vi "UI_visual2.vi"() -> ()   [LabVIEW 2017]
uses:
  <vilib>/picture/3D Picture Control/NI_3D Picture Control.lvlib
  <vilib>/picture/3D Picture Control/Object/Add Object (no reference).vi
  <vilib>/Utility/miscctls.llb/LV3DPointTypeDef.ctl
  <vilib>/Analysis/coordinate.llb/Euler Rotation Order.ctl
  <vilib>/Analysis/NI_AALPro.lvlib
  <vilib>/picture/3D Picture Control/Object/Create Object (name).vi
  <vilib>/picture/3D Picture Control/Helpers/Apply Texture (no reference).vi
  <vilib>/picture/3D Picture Control/Helpers/Set Clip Plane (no reference).vi
panel:
  out "element":dbl
  in  "Simulation Parameters":T1={"Wind VelocityAzimuth [deg] "=0.0, "Wind Velocity Module [m/s]"=0.0, "Fe gain"=1.0, "Cnalpha gain"=1.0, "clp gain"=1.0, "cld gain"=1.0, "cmq gain"=1.0, "cnr gain"=1.0, "dl [º]"=0.0, "Nozzle misalignment yaw/pitch [º]"=[0.0, 0.0], "Nozzle eccentricity x/y [m]"=[], "Wind_Profile"=0} {"Wind_Profile" min=0 max=3 step=1; "Wind Velocity Module [m/s]" format="%#_13g"; "Wind VelocityAzimuth [deg]" format="%#_13g"}
  in  "Initialization Parameters":T2={"W_b ini [rad/s]"=[0.0, 0.0, 0.0], "W ini [rad/s]"=[0.0, 0.0, 0.0], "altitude_ini(m)"=50.0, "lon_ini [º]"=-44.36778, "latd_ini [º]"=-2.31599, "V_ini [m/s]"=[0.0, 0.0, 0.0], "Initial Euler Angles [deg]"=[0.0, 0.0, 0.0], "CFN-61G Enable"=FALSE, "Table enable"=FALSE, "DMARS Enable"=FALSE, "TVA Enable"=FALSE, "Sim_Time [s]"=82.0}
  out "CRC data fault":bool
  out "Euler Angles [rad]":dbl[](array[numeric])
  in  "Tab Control":T3(tab)
  out "Position":cluster{dbl[], dbl[]}[](graph)
  out "Velocity":cluster{dbl[], dbl[]}[](graph)
  out "Quaternions":cluster{dbl[], dbl[]}[](graph)
  out "Euler Angles":cluster{dbl[], dbl[]}[](graph)
  out "Body Rates":cluster{dbl[], dbl[]}[](graph)
  out "Body Accelerations":cluster{dbl[], dbl[]}[](graph)
  out "Malpha/ Mbeta":cluster{dbl[], dbl[]}[](graph)
  out "Angles of attack":cluster{dbl[], dbl[]}[](graph)
  out "ACT_b_angles":cluster{dbl[], dbl[]}[](graph)
  out "Oil Consumption":cluster{dbl[], dbl[]}(graph)
  out "Bending Moments":dbl[](graph)
  out "CRC Failures":cluster{dbl[], dbl[]}[](graph)
  out "Euler Angles 2":cluster{dbl[], dbl[]}[](graph)
  out "Sim_Stopped":bool
  in  "stop Host":bool
  in  "Run_SIM":bool
  out "time[s]":dbl
  out "Euler Angles [º]":dbl[](array[numeric])
  out "B-frame [m]":cluster{"X":sgl, "Y":sgl, "Z":sgl}
  in  "B-frame Translation 2":cluster{"X":sgl, "Y":sgl, "Z":sgl}
  in  "N-frame rot":dbl[](array[numeric])
  in  "Up Direction":T4={"X"=0.0, "Y"=0.0, "Z"=1.0}
  out "3D Picture Control":refnum<vi>(3d-picture)
  in  "error in (no error)":errorcluster
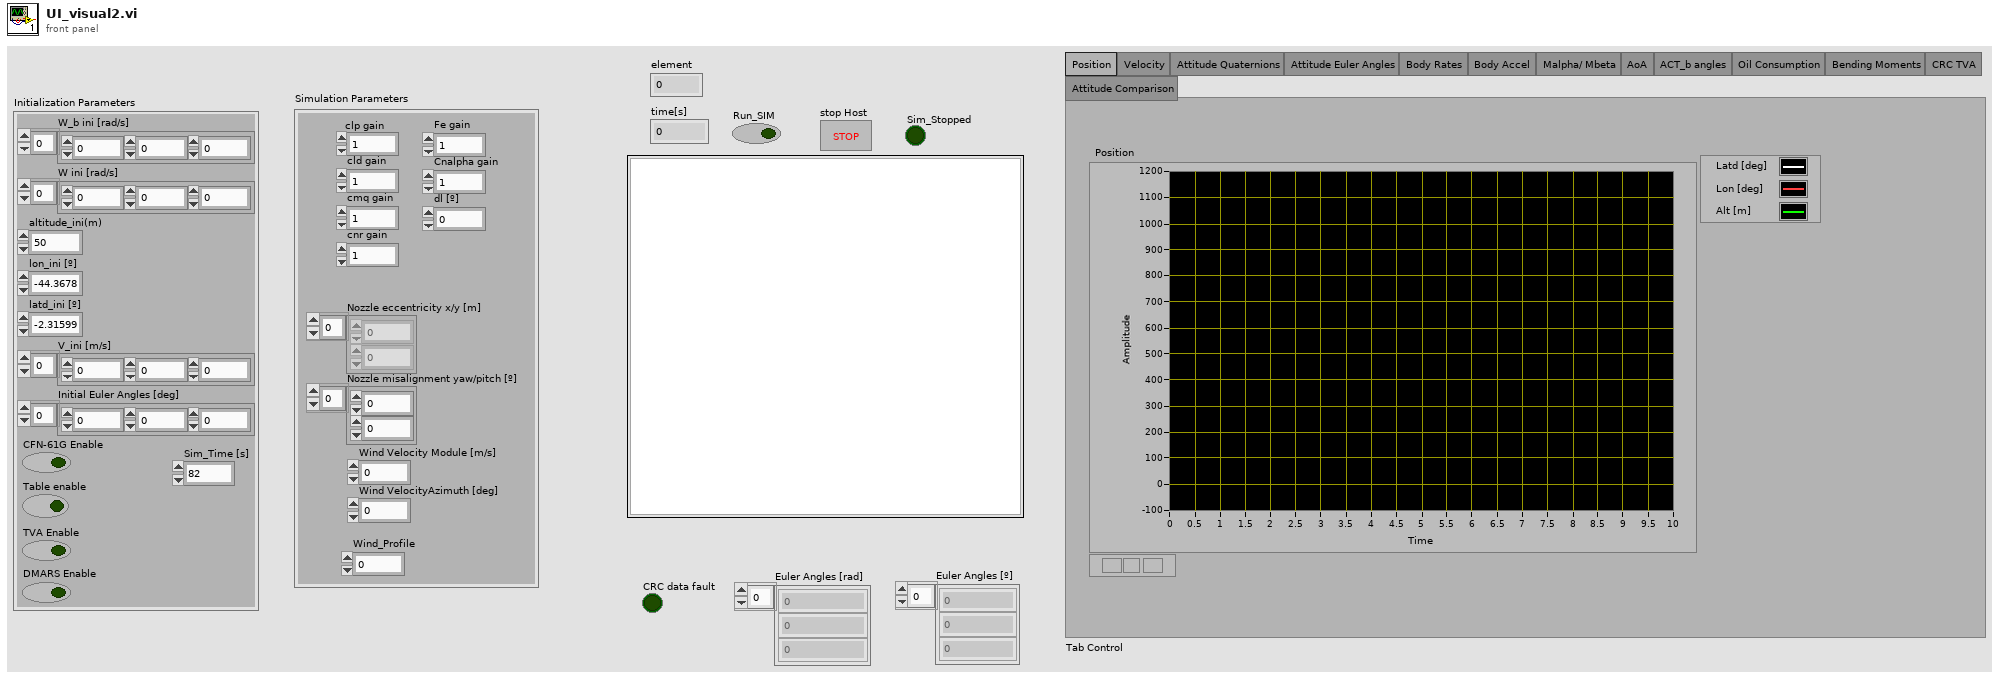
[diagram p1: front panel]
types:
  T1 = cluster{"Wind VelocityAzimuth [deg] ":dbl, "Wind Velocity Module [m/s]":dbl, "Fe gain":dbl, "Cnalpha gain":dbl, "clp gain":dbl, "cld gain":dbl, "cmq gain":dbl, "cnr gain":dbl, "dl [º]":dbl, "Nozzle misalignment yaw/pitch [º]":dbl[], "Nozzle eccentricity x/y [m]":dbl[], "Wind_Profile":i32}
  T2 = cluster{"W_b ini [rad/s]":dbl[], "W ini [rad/s]":dbl[], "altitude_ini(m)":dbl, "lon_ini [º]":dbl, "latd_ini [º]":dbl, "V_ini [m/s]":dbl[], "Initial Euler Angles [deg]":dbl[], "CFN-61G Enable":bool, "Table enable":bool, "DMARS Enable":bool, "TVA Enable":bool, "Sim_Time [s]":dbl}
  T3 = enum32{"Position", "Velocity", "Attitude Quaternions", "Attitude Euler Angles", "Body Rates", "Body Accel", "Malpha/ Mbeta", "AoA", "ACT_b angles", "Oil Consumption", "Bending Moments", "CRC TVA", "Attitude Comparison"}
  T4 = typedef "LV3DPointTypeDef.ctl" = cluster{"X":sgl, "Y":sgl, "Z":sgl}
  T5 = enum16{"As a Decal", "With Modulation", "With Blending", "As a replacement"}
  T6 = cluster{"Red":sgl, "Green":sgl, "Blue":sgl, "Alpha":sgl}
  T7 = typedef "NI_AALPro.lvlib/Euler Rotation Order.ctl" = u16
  T8 = typedef "imagedata.ctl" = cluster{"image type":i32, "image depth":i32, "image":u8[], "mask":u8[], "colors":u32[], "Rectangle":cluster{"left":i16, "top":i16, "right":i16, "bottom":i16}}
  T9 = cluster{"element":dbl, "element":dbl, "element":dbl}
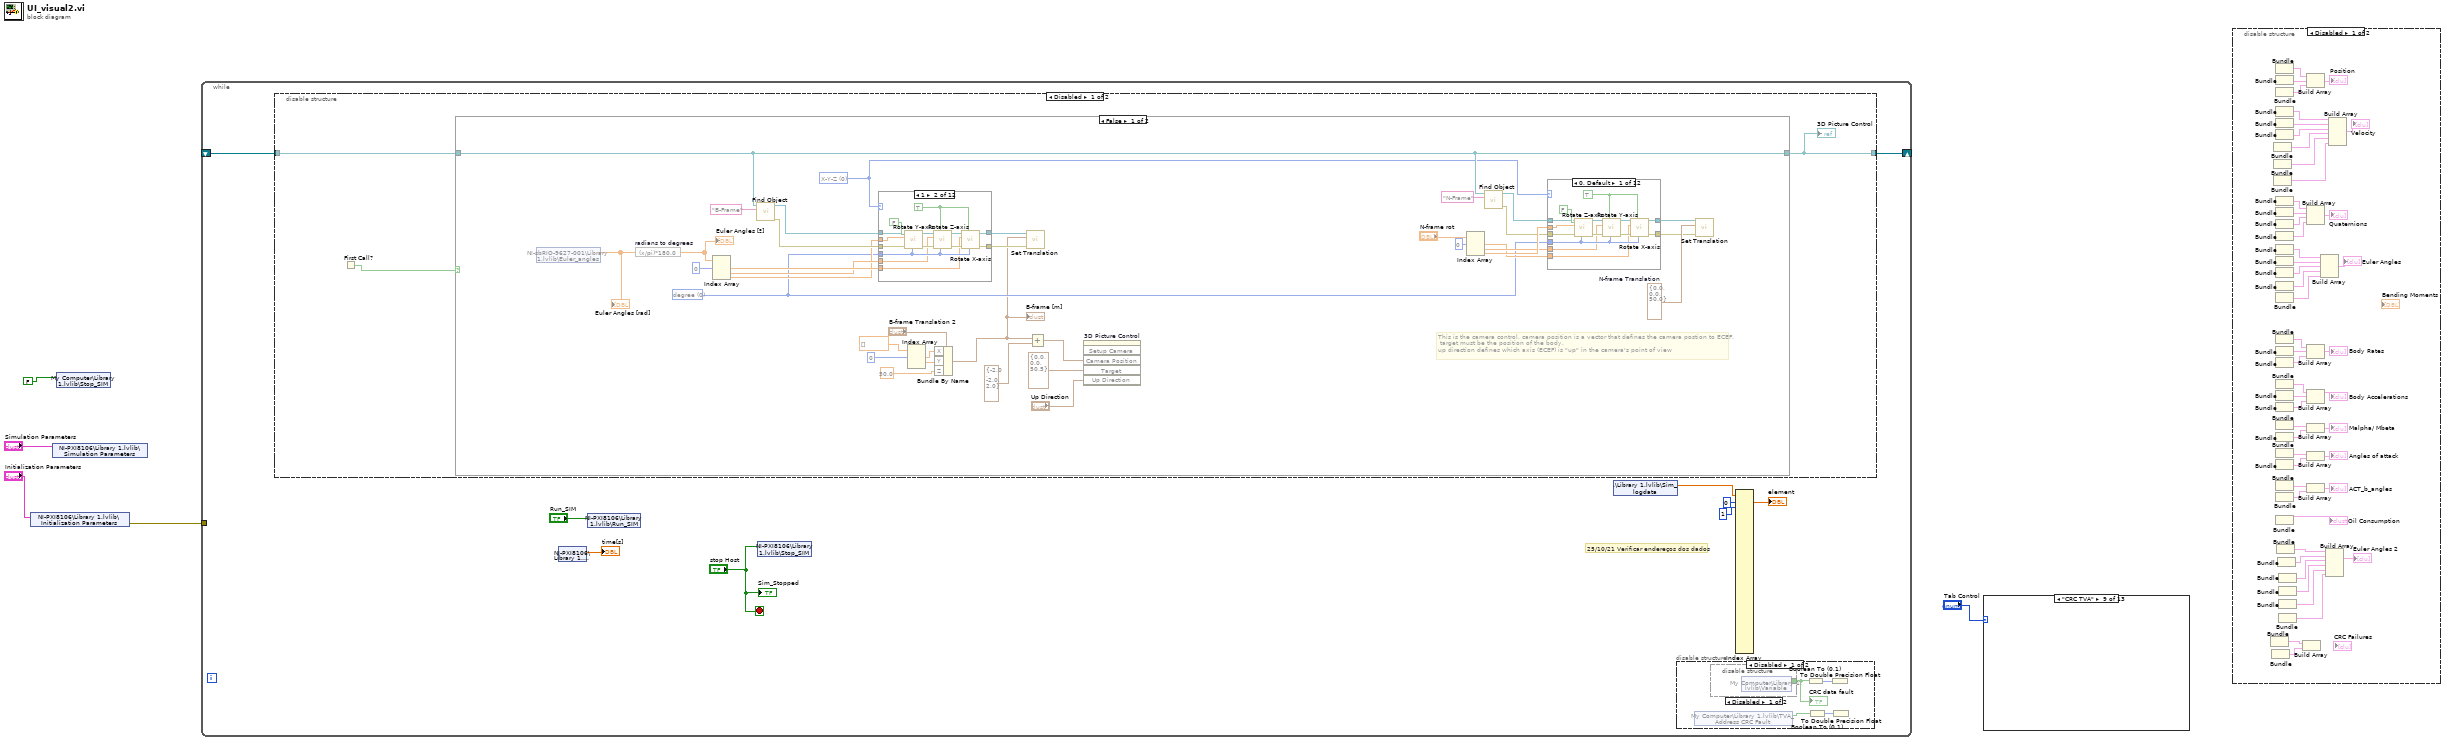
[diagram p0: block diagram]
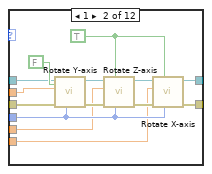
[diagram p17: hidden frame]
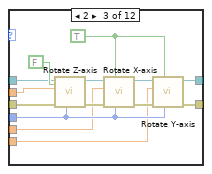
[diagram p18: hidden frame]
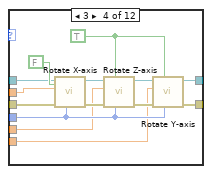
[diagram p19: hidden frame]
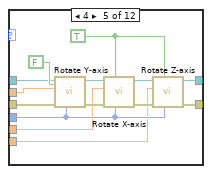
[diagram p20: hidden frame]
diagram:
  n1 = shared-variable "NI-PXI8106\\Library 1.lvlib\\Initialization Parameters"("Initialization Parameters") -> (error out=w1:errorcluster)  [unwired: 1 in]
  n2 = shared-variable "NI-PXI8106\\Library 1.lvlib\\Simulation Parameters"("Simulation Parameters") -> ()  [unwired: 1 in, 1 out]
  n3 = shared-variable "My Computer\\Library 1.lvlib\\Stop_SIM"(FALSE) -> ()  [unwired: 1 in, 1 out]
  n4 = while {
    shift-right: [w13] -> _
    shift-left: _ -> [w14]
    tunnel: w1 -> [_]
    stop <- "stop Host" stop-if-true
    # "25/10/21 Verificar endereços dos dados"
    n5 = disable-structure shown="Disabled" {
      disable-tunnel: w14 -> [w22 _]
      disable-tunnel: [w21 _] -> w13
      frame Disabled {
        n6 = First Call?() -> (First Call?: T/F=w20:bool)
        n7 = case shown="False" w20 {
          tunnel: [w39 w402] -> w21
          tunnel: w22 -> [w39 _]
          frame False {
            w38 = T7 0 items=["X-Y-Z", "X-Z-Y", "Y-X-Z", "Y-Z-X", "Z-X-Y", "Z-Y-X", "X-Y-X", "X-Z-X", "Y-X-Y", "Y-Z-Y", "Z-X-Z", "Z-Y-Z"] ("rotation order")
            w49 = cluster{"X":sgl, "Y":sgl, "Z":sgl} {"X"=0.0, "Y"=0.0, "Z"=50.0}  # N-frame Translation
            w37 = u16 0 items=["degree", "radians"] ("angle unit")
            # "This is the camera control, camera position is a vector that defines the camera postion to ECEF,\n target must be the position of the body. \nup direction defines which axis (ECEF) is \"up\" in the camera's point of view"
            n8 = shared-variable "NI-sbRIO-9627-001\\Library 1.lvlib\\Euler_angles"() -> (w31:dbl[])  [unwired: 1 in, 1 out]
            "Euler Angles [rad]" <- w31
            n9 = expression code="(x/pi)*180.0" "radians to degrees"(w31) -> (w32:dbl[])
            "Euler Angles [º]" <- w32
            n10 = Index Array(array=w32, index #1=0 ("index")) -> (element #1=w57:dbl, element #2=w54:dbl, element #3=w53:dbl)  [unwired: 2 in]
            n11 = call <vilib>:"Find Object.vi"("Object Name"="B-Frame", "Scene Refnum"=w39) -> ("error out"=w55:errorcluster, "Object Refnum"=w56:refnum<vi>)  [unwired: 8 in]
            n12 = case shown="1" w38 {
              tunnel: w57 -> [w231 w247 w261 w275 w285 w303 w317 w331 w345 w356 w370 w384]
              tunnel: w56 -> [w234 w244 w257 w271 w289 w299 w316 w330 w341 w360 w374 w388]
              tunnel: w55 -> [w233 w243 w258 w272 w288 w300 w315 w329 w342 w359 w373 w387]
              tunnel: w54 -> [w230 w245 w260 w274 w286 w302 w313 w327 w344 w357 w371 w386]
              tunnel: w53 -> [w229 w246 w259 w273 w287 w301 w314 w328 w343 w358 w372 w385]
              tunnel: w37 -> [w232 w248 w262 w276 w290 w304 w318 w332 w346 w355 w369 w383]
              tunnel: [w228 w242 w256 w270 w284 w298 w312 w326 w340 w354 w368 w382] -> w51
              tunnel: [w227 w241 w255 w269 w283 w297 w311 w325 w339 w353 w367 w381] -> w50
              frame 0, Default {
                w240 = TRUE ("Relative?")
                n13 = call <vilib>:"Rotate Z-axis.vi"("angle unit"=w232, "Relative?"=FALSE, "error in (no error)"=w233, "angle"=w229, "Scene Object In"=w234) -> ("error out"=w237:errorcluster, "Scene Object Out"=w238:refnum<vi>)  [unwired: 5 in]
                n14 = call <vilib>:"Rotate Y-axis.vi"("angle unit"=w232, "Relative?"=w240, "error in (no error)"=w237, "angle"=w230, "Scene Object In"=w238) -> ("error out"=w236:errorcluster, "Scene Object Out"=w235:refnum<vi>)  [unwired: 5 in]
                n15 = call <vilib>:"Rotate X-axis.vi"("angle unit"=w232, "Relative?"=w240, "error in (no error)"=w236, "angle"=w231, "Scene Object In"=w235) -> ("error out"=w227:errorcluster, "Scene Object Out"=w228:refnum<vi>)  [unwired: 5 in]
              }
              frame 1 {
                w251 = TRUE ("Relative?")
                n16 = call <vilib>:"Rotate Y-axis.vi"("angle unit"=w248, "Relative?"=FALSE, "error in (no error)"=w243, "angle"=w246, "Scene Object In"=w244) -> ("error out"=w252:errorcluster, "Scene Object Out"=w253:refnum<vi>)  [unwired: 5 in]
                n17 = call <vilib>:"Rotate Z-axis.vi"("angle unit"=w248, "Relative?"=w251, "error in (no error)"=w252, "angle"=w245, "Scene Object In"=w253) -> ("error out"=w249:errorcluster, "Scene Object Out"=w250:refnum<vi>)  [unwired: 5 in]
                n18 = call <vilib>:"Rotate X-axis.vi"("angle unit"=w248, "Relative?"=w251, "error in (no error)"=w249, "angle"=w247, "Scene Object In"=w250) -> ("error out"=w241:errorcluster, "Scene Object Out"=w242:refnum<vi>)  [unwired: 5 in]
              }
              frame 2 {
                w263 = TRUE ("Relative?")
                n19 = call <vilib>:"Rotate Z-axis.vi"("angle unit"=w262, "Relative?"=FALSE, "error in (no error)"=w258, "angle"=w259, "Scene Object In"=w257) -> ("error out"=w266:errorcluster, "Scene Object Out"=w267:refnum<vi>)  [unwired: 5 in]
                n20 = call <vilib>:"Rotate X-axis.vi"("angle unit"=w262, "Relative?"=w263, "error in (no error)"=w266, "angle"=w260, "Scene Object In"=w267) -> ("error out"=w264:errorcluster, "Scene Object Out"=w265:refnum<vi>)  [unwired: 5 in]
                n21 = call <vilib>:"Rotate Y-axis.vi"("angle unit"=w262, "Relative?"=w263, "error in (no error)"=w264, "angle"=w261, "Scene Object In"=w265) -> ("error out"=w255:errorcluster, "Scene Object Out"=w256:refnum<vi>)  [unwired: 5 in]
              }
              frame 3 {
                w281 = TRUE ("Relative?")
                n22 = call <vilib>:"Rotate X-axis.vi"("angle unit"=w276, "Relative?"=FALSE, "error in (no error)"=w272, "angle"=w273, "Scene Object In"=w271) -> ("error out"=w279:errorcluster, "Scene Object Out"=w280:refnum<vi>)  [unwired: 5 in]
                n23 = call <vilib>:"Rotate Z-axis.vi"("angle unit"=w276, "Relative?"=w281, "error in (no error)"=w279, "angle"=w274, "Scene Object In"=w280) -> ("error out"=w277:errorcluster, "Scene Object Out"=w278:refnum<vi>)  [unwired: 5 in]
                n24 = call <vilib>:"Rotate Y-axis.vi"("angle unit"=w276, "Relative?"=w281, "error in (no error)"=w277, "angle"=w275, "Scene Object In"=w278) -> ("error out"=w269:errorcluster, "Scene Object Out"=w270:refnum<vi>)  [unwired: 5 in]
              }
              frame 4 {
                w295 = TRUE ("Relative?")
                n25 = call <vilib>:"Rotate Y-axis.vi"("angle unit"=w290, "Relative?"=FALSE, "error in (no error)"=w288, "angle"=w287, "Scene Object In"=w289) -> ("error out"=w291:errorcluster, "Scene Object Out"=w292:refnum<vi>)  [unwired: 5 in]
                n26 = call <vilib>:"Rotate X-axis.vi"("angle unit"=w290, "Relative?"=w295, "error in (no error)"=w291, "angle"=w286, "Scene Object In"=w292) -> ("error out"=w294:errorcluster, "Scene Object Out"=w293:refnum<vi>)  [unwired: 5 in]
                n27 = call <vilib>:"Rotate Z-axis.vi"("angle unit"=w290, "Relative?"=w295, "error in (no error)"=w294, "angle"=w285, "Scene Object In"=w293) -> ("error out"=w283:errorcluster, "Scene Object Out"=w284:refnum<vi>)  [unwired: 5 in]
              }
              frame 5 {
                w308 = TRUE ("Relative?")
                n28 = call <vilib>:"Rotate X-axis.vi"("angle unit"=w304, "Relative?"=FALSE, "error in (no error)"=w300, "angle"=w301, "Scene Object In"=w299) -> ("error out"=w306:errorcluster, "Scene Object Out"=w307:refnum<vi>)  [unwired: 5 in]
                n29 = call <vilib>:"Rotate Y-axis.vi"("angle unit"=w304, "Relative?"=w308, "error in (no error)"=w306, "angle"=w302, "Scene Object In"=w307) -> ("error out"=w310:errorcluster, "Scene Object Out"=w309:refnum<vi>)  [unwired: 5 in]
                n30 = call <vilib>:"Rotate Z-axis.vi"("angle unit"=w304, "Relative?"=w308, "error in (no error)"=w310, "angle"=w303, "Scene Object In"=w309) -> ("error out"=w297:errorcluster, "Scene Object Out"=w298:refnum<vi>)  [unwired: 5 in]
              }
              frame 6 {
                w321 = TRUE ("Relative?")
                n31 = call <vilib>:"Rotate X-axis.vi"("angle unit"=w318, "Relative?"=FALSE, "error in (no error)"=w315, "angle"=w314, "Scene Object In"=w316) -> ("error out"=w323:errorcluster, "Scene Object Out"=w324:refnum<vi>)  [unwired: 5 in]
                n32 = call <vilib>:"Rotate Y-axis.vi"("angle unit"=w318, "Relative?"=w321, "error in (no error)"=w323, "angle"=w313, "Scene Object In"=w324) -> ("error out"=w319:errorcluster, "Scene Object Out"=w320:refnum<vi>)  [unwired: 5 in]
                n33 = call <vilib>:"Rotate X-axis.vi"("angle unit"=w318, "Relative?"=w321, "error in (no error)"=w319, "angle"=w317, "Scene Object In"=w320) -> ("error out"=w311:errorcluster, "Scene Object Out"=w312:refnum<vi>)  [unwired: 5 in]
              }
              frame 7 {
                w337 = TRUE ("Relative?")
                n34 = call <vilib>:"Rotate X-axis.vi"("angle unit"=w332, "Relative?"=FALSE, "error in (no error)"=w329, "angle"=w328, "Scene Object In"=w330) -> ("error out"=w335:errorcluster, "Scene Object Out"=w336:refnum<vi>)  [unwired: 5 in]
                n35 = call <vilib>:"Rotate Z-axis.vi"("angle unit"=w332, "Relative?"=w337, "error in (no error)"=w335, "angle"=w327, "Scene Object In"=w336) -> ("error out"=w334:errorcluster, "Scene Object Out"=w333:refnum<vi>)  [unwired: 5 in]
                n36 = call <vilib>:"Rotate X-axis.vi"("angle unit"=w332, "Relative?"=w337, "error in (no error)"=w334, "angle"=w331, "Scene Object In"=w333) -> ("error out"=w325:errorcluster, "Scene Object Out"=w326:refnum<vi>)  [unwired: 5 in]
              }
              frame 8 {
                w351 = TRUE ("Relative?")
                n37 = call <vilib>:"Rotate Y-axis.vi"("angle unit"=w346, "Relative?"=FALSE, "error in (no error)"=w342, "angle"=w343, "Scene Object In"=w341) -> ("error out"=w349:errorcluster, "Scene Object Out"=w350:refnum<vi>)  [unwired: 5 in]
                n38 = call <vilib>:"Rotate X-axis.vi"("angle unit"=w346, "Relative?"=w351, "error in (no error)"=w349, "angle"=w344, "Scene Object In"=w350) -> ("error out"=w348:errorcluster, "Scene Object Out"=w347:refnum<vi>)  [unwired: 5 in]
                n39 = call <vilib>:"Rotate Y-axis.vi"("angle unit"=w346, "Relative?"=w351, "error in (no error)"=w348, "angle"=w345, "Scene Object In"=w347) -> ("error out"=w339:errorcluster, "Scene Object Out"=w340:refnum<vi>)  [unwired: 5 in]
              }
              frame 9 {
                w365 = TRUE ("Relative?")
                n40 = call <vilib>:"Rotate Y-axis.vi"("angle unit"=w355, "Relative?"=FALSE, "error in (no error)"=w359, "angle"=w358, "Scene Object In"=w360) -> ("error out"=w363:errorcluster, "Scene Object Out"=w364:refnum<vi>)  [unwired: 5 in]
                n41 = call <vilib>:"Rotate Z-axis.vi"("angle unit"=w355, "Relative?"=w365, "error in (no error)"=w363, "angle"=w357, "Scene Object In"=w364) -> ("error out"=w362:errorcluster, "Scene Object Out"=w361:refnum<vi>)  [unwired: 5 in]
                n42 = call <vilib>:"Rotate Y-axis.vi"("angle unit"=w355, "Relative?"=w365, "error in (no error)"=w362, "angle"=w356, "Scene Object In"=w361) -> ("error out"=w353:errorcluster, "Scene Object Out"=w354:refnum<vi>)  [unwired: 5 in]
              }
              frame 10 {
                w379 = TRUE ("Relative?")
                n43 = call <vilib>:"Rotate Z-axis.vi"("angle unit"=w369, "Relative?"=FALSE, "error in (no error)"=w373, "angle"=w372, "Scene Object In"=w374) -> ("error out"=w377:errorcluster, "Scene Object Out"=w378:refnum<vi>)  [unwired: 5 in]
                n44 = call <vilib>:"Rotate X-axis.vi"("angle unit"=w369, "Relative?"=w379, "error in (no error)"=w377, "angle"=w371, "Scene Object In"=w378) -> ("error out"=w376:errorcluster, "Scene Object Out"=w375:refnum<vi>)  [unwired: 5 in]
                n45 = call <vilib>:"Rotate Z-axis.vi"("angle unit"=w369, "Relative?"=w379, "error in (no error)"=w376, "angle"=w370, "Scene Object In"=w375) -> ("error out"=w367:errorcluster, "Scene Object Out"=w368:refnum<vi>)  [unwired: 5 in]
              }
              frame 11 {
                w393 = TRUE ("Relative?")
                n46 = call <vilib>:"Rotate Z-axis.vi"("angle unit"=w383, "Relative?"=FALSE, "error in (no error)"=w387, "angle"=w385, "Scene Object In"=w388) -> ("error out"=w391:errorcluster, "Scene Object Out"=w392:refnum<vi>)  [unwired: 5 in]
                n47 = call <vilib>:"Rotate Y-axis.vi"("angle unit"=w383, "Relative?"=w393, "error in (no error)"=w391, "angle"=w386, "Scene Object In"=w392) -> ("error out"=w390:errorcluster, "Scene Object Out"=w389:refnum<vi>)  [unwired: 5 in]
                n48 = call <vilib>:"Rotate Z-axis.vi"("angle unit"=w383, "Relative?"=w393, "error in (no error)"=w390, "angle"=w384, "Scene Object In"=w389) -> ("error out"=w381:errorcluster, "Scene Object Out"=w382:refnum<vi>)  [unwired: 5 in]
              }
            }
            n49 = Index Array(array=dbl[] [], index #1=0 ("index")) -> (element #1=w34:dbl, element #2=w33:dbl)  [unwired: 2 in, 1 out]
            n50 = Bundle By Name(cluster="B-frame Translation 2", "X"=w34, "Y"=w33, "Z"=50.0 ("Double")) -> (w25:cluster{"X":sgl, "Y":sgl, "Z":sgl})
            "B-frame [m]" <- w25
            n51 = call <vilib>:"Set Translation.vi"("error in (no error)"=w50, "Translation"=w25, "Scene Object"=w51) -> ()  [unwired: 7 in, 2 out]
            n52 = Add(x=w25, y=T4 {"X"=-2.0, "Y"=-2.0, "Z"=2.0} ("Camera Position control")) -> (x+y=w26:T4)
            n53 = invoke on="3D Picture Control" class="SceneGraphDisp (strict)" method="Setup Camera"("Camera Position"=w26, "Target"=T4 {"X"=0.0, "Y"=0.0, "Z"=50.5}, "Up Direction"="Up Direction") -> ()  [unwired: 3 in, 6 out]
            n54 = Index Array(array="N-frame rot", index #1=0 ("index")) -> (element #1=w41:dbl, element #2=w44:dbl, element #3=w45:dbl)  [unwired: 2 in]
            n55 = call <vilib>:"Find Object.vi"("Object Name"="N-Frame", "Scene Refnum"=w39) -> ("error out"=w43:errorcluster, "Object Refnum"=w42:refnum<vi>)  [unwired: 8 in]
            n56 = case shown="0, Default" w38 {
              tunnel: w41 -> [w63 w79 w93 w107 w117 w135 w149 w163 w177 w188 w202 w216]
              tunnel: w42 -> [w66 w76 w89 w103 w121 w131 w148 w162 w173 w192 w206 w220]
              tunnel: w43 -> [w65 w75 w90 w104 w120 w132 w147 w161 w174 w191 w205 w219]
              tunnel: w44 -> [w62 w77 w92 w106 w118 w134 w145 w159 w176 w189 w203 w218]
              tunnel: w45 -> [w61 w78 w91 w105 w119 w133 w146 w160 w175 w190 w204 w217]
              tunnel: w37 -> [w64 w80 w94 w108 w122 w136 w150 w164 w178 w187 w201 w215]
              tunnel: [w60 w74 w88 w102 w116 w130 w144 w158 w172 w186 w200 w214] -> w47
              tunnel: [w59 w73 w87 w101 w115 w129 w143 w157 w171 w185 w199 w213] -> w48
              frame 0, Default {
                w72 = TRUE ("Relative?")
                n57 = call <vilib>:"Rotate Z-axis.vi"("angle unit"=w64, "Relative?"=FALSE, "error in (no error)"=w65, "angle"=w61, "Scene Object In"=w66) -> ("error out"=w69:errorcluster, "Scene Object Out"=w70:refnum<vi>)  [unwired: 5 in]
                n58 = call <vilib>:"Rotate Y-axis.vi"("angle unit"=w64, "Relative?"=w72, "error in (no error)"=w69, "angle"=w62, "Scene Object In"=w70) -> ("error out"=w68:errorcluster, "Scene Object Out"=w67:refnum<vi>)  [unwired: 5 in]
                n59 = call <vilib>:"Rotate X-axis.vi"("angle unit"=w64, "Relative?"=w72, "error in (no error)"=w68, "angle"=w63, "Scene Object In"=w67) -> ("error out"=w59:errorcluster, "Scene Object Out"=w60:refnum<vi>)  [unwired: 5 in]
              }
              frame 1 {
                w83 = TRUE ("Relative?")
                n60 = call <vilib>:"Rotate Y-axis.vi"("angle unit"=w80, "Relative?"=FALSE, "error in (no error)"=w75, "angle"=w78, "Scene Object In"=w76) -> ("error out"=w84:errorcluster, "Scene Object Out"=w85:refnum<vi>)  [unwired: 5 in]
                n61 = call <vilib>:"Rotate Z-axis.vi"("angle unit"=w80, "Relative?"=w83, "error in (no error)"=w84, "angle"=w77, "Scene Object In"=w85) -> ("error out"=w81:errorcluster, "Scene Object Out"=w82:refnum<vi>)  [unwired: 5 in]
                n62 = call <vilib>:"Rotate X-axis.vi"("angle unit"=w80, "Relative?"=w83, "error in (no error)"=w81, "angle"=w79, "Scene Object In"=w82) -> ("error out"=w73:errorcluster, "Scene Object Out"=w74:refnum<vi>)  [unwired: 5 in]
              }
              frame 2 {
                w95 = TRUE ("Relative?")
                n63 = call <vilib>:"Rotate Z-axis.vi"("angle unit"=w94, "Relative?"=FALSE, "error in (no error)"=w90, "angle"=w91, "Scene Object In"=w89) -> ("error out"=w98:errorcluster, "Scene Object Out"=w99:refnum<vi>)  [unwired: 5 in]
                n64 = call <vilib>:"Rotate X-axis.vi"("angle unit"=w94, "Relative?"=w95, "error in (no error)"=w98, "angle"=w92, "Scene Object In"=w99) -> ("error out"=w96:errorcluster, "Scene Object Out"=w97:refnum<vi>)  [unwired: 5 in]
                n65 = call <vilib>:"Rotate Y-axis.vi"("angle unit"=w94, "Relative?"=w95, "error in (no error)"=w96, "angle"=w93, "Scene Object In"=w97) -> ("error out"=w87:errorcluster, "Scene Object Out"=w88:refnum<vi>)  [unwired: 5 in]
              }
              frame 3 {
                w113 = TRUE ("Relative?")
                n66 = call <vilib>:"Rotate X-axis.vi"("angle unit"=w108, "Relative?"=FALSE, "error in (no error)"=w104, "angle"=w105, "Scene Object In"=w103) -> ("error out"=w111:errorcluster, "Scene Object Out"=w112:refnum<vi>)  [unwired: 5 in]
                n67 = call <vilib>:"Rotate Z-axis.vi"("angle unit"=w108, "Relative?"=w113, "error in (no error)"=w111, "angle"=w106, "Scene Object In"=w112) -> ("error out"=w109:errorcluster, "Scene Object Out"=w110:refnum<vi>)  [unwired: 5 in]
                n68 = call <vilib>:"Rotate Y-axis.vi"("angle unit"=w108, "Relative?"=w113, "error in (no error)"=w109, "angle"=w107, "Scene Object In"=w110) -> ("error out"=w101:errorcluster, "Scene Object Out"=w102:refnum<vi>)  [unwired: 5 in]
              }
              frame 4 {
                w127 = TRUE ("Relative?")
                n69 = call <vilib>:"Rotate Y-axis.vi"("angle unit"=w122, "Relative?"=FALSE, "error in (no error)"=w120, "angle"=w119, "Scene Object In"=w121) -> ("error out"=w123:errorcluster, "Scene Object Out"=w124:refnum<vi>)  [unwired: 5 in]
                n70 = call <vilib>:"Rotate X-axis.vi"("angle unit"=w122, "Relative?"=w127, "error in (no error)"=w123, "angle"=w118, "Scene Object In"=w124) -> ("error out"=w126:errorcluster, "Scene Object Out"=w125:refnum<vi>)  [unwired: 5 in]
                n71 = call <vilib>:"Rotate Z-axis.vi"("angle unit"=w122, "Relative?"=w127, "error in (no error)"=w126, "angle"=w117, "Scene Object In"=w125) -> ("error out"=w115:errorcluster, "Scene Object Out"=w116:refnum<vi>)  [unwired: 5 in]
              }
              frame 5 {
                w140 = TRUE ("Relative?")
                n72 = call <vilib>:"Rotate X-axis.vi"("angle unit"=w136, "Relative?"=FALSE, "error in (no error)"=w132, "angle"=w133, "Scene Object In"=w131) -> ("error out"=w138:errorcluster, "Scene Object Out"=w139:refnum<vi>)  [unwired: 5 in]
                n73 = call <vilib>:"Rotate Y-axis.vi"("angle unit"=w136, "Relative?"=w140, "error in (no error)"=w138, "angle"=w134, "Scene Object In"=w139) -> ("error out"=w142:errorcluster, "Scene Object Out"=w141:refnum<vi>)  [unwired: 5 in]
                n74 = call <vilib>:"Rotate Z-axis.vi"("angle unit"=w136, "Relative?"=w140, "error in (no error)"=w142, "angle"=w135, "Scene Object In"=w141) -> ("error out"=w129:errorcluster, "Scene Object Out"=w130:refnum<vi>)  [unwired: 5 in]
              }
              frame 6 {
                w153 = TRUE ("Relative?")
                n75 = call <vilib>:"Rotate X-axis.vi"("angle unit"=w150, "Relative?"=FALSE, "error in (no error)"=w147, "angle"=w146, "Scene Object In"=w148) -> ("error out"=w155:errorcluster, "Scene Object Out"=w156:refnum<vi>)  [unwired: 5 in]
                n76 = call <vilib>:"Rotate Y-axis.vi"("angle unit"=w150, "Relative?"=w153, "error in (no error)"=w155, "angle"=w145, "Scene Object In"=w156) -> ("error out"=w151:errorcluster, "Scene Object Out"=w152:refnum<vi>)  [unwired: 5 in]
                n77 = call <vilib>:"Rotate X-axis.vi"("angle unit"=w150, "Relative?"=w153, "error in (no error)"=w151, "angle"=w149, "Scene Object In"=w152) -> ("error out"=w143:errorcluster, "Scene Object Out"=w144:refnum<vi>)  [unwired: 5 in]
              }
              frame 7 {
                w169 = TRUE ("Relative?")
                n78 = call <vilib>:"Rotate X-axis.vi"("angle unit"=w164, "Relative?"=FALSE, "error in (no error)"=w161, "angle"=w160, "Scene Object In"=w162) -> ("error out"=w167:errorcluster, "Scene Object Out"=w168:refnum<vi>)  [unwired: 5 in]
                n79 = call <vilib>:"Rotate Z-axis.vi"("angle unit"=w164, "Relative?"=w169, "error in (no error)"=w167, "angle"=w159, "Scene Object In"=w168) -> ("error out"=w166:errorcluster, "Scene Object Out"=w165:refnum<vi>)  [unwired: 5 in]
                n80 = call <vilib>:"Rotate X-axis.vi"("angle unit"=w164, "Relative?"=w169, "error in (no error)"=w166, "angle"=w163, "Scene Object In"=w165) -> ("error out"=w157:errorcluster, "Scene Object Out"=w158:refnum<vi>)  [unwired: 5 in]
              }
              frame 8 {
                w183 = TRUE ("Relative?")
                n81 = call <vilib>:"Rotate Y-axis.vi"("angle unit"=w178, "Relative?"=FALSE, "error in (no error)"=w174, "angle"=w175, "Scene Object In"=w173) -> ("error out"=w181:errorcluster, "Scene Object Out"=w182:refnum<vi>)  [unwired: 5 in]
                n82 = call <vilib>:"Rotate X-axis.vi"("angle unit"=w178, "Relative?"=w183, "error in (no error)"=w181, "angle"=w176, "Scene Object In"=w182) -> ("error out"=w180:errorcluster, "Scene Object Out"=w179:refnum<vi>)  [unwired: 5 in]
                n83 = call <vilib>:"Rotate Y-axis.vi"("angle unit"=w178, "Relative?"=w183, "error in (no error)"=w180, "angle"=w177, "Scene Object In"=w179) -> ("error out"=w171:errorcluster, "Scene Object Out"=w172:refnum<vi>)  [unwired: 5 in]
              }
              frame 9 {
                w197 = TRUE ("Relative?")
                n84 = call <vilib>:"Rotate Y-axis.vi"("angle unit"=w187, "Relative?"=FALSE, "error in (no error)"=w191, "angle"=w190, "Scene Object In"=w192) -> ("error out"=w195:errorcluster, "Scene Object Out"=w196:refnum<vi>)  [unwired: 5 in]
                n85 = call <vilib>:"Rotate Z-axis.vi"("angle unit"=w187, "Relative?"=w197, "error in (no error)"=w195, "angle"=w189, "Scene Object In"=w196) -> ("error out"=w194:errorcluster, "Scene Object Out"=w193:refnum<vi>)  [unwired: 5 in]
                n86 = call <vilib>:"Rotate Y-axis.vi"("angle unit"=w187, "Relative?"=w197, "error in (no error)"=w194, "angle"=w188, "Scene Object In"=w193) -> ("error out"=w185:errorcluster, "Scene Object Out"=w186:refnum<vi>)  [unwired: 5 in]
              }
              frame 10 {
                w211 = TRUE ("Relative?")
                n87 = call <vilib>:"Rotate Z-axis.vi"("angle unit"=w201, "Relative?"=FALSE, "error in (no error)"=w205, "angle"=w204, "Scene Object In"=w206) -> ("error out"=w209:errorcluster, "Scene Object Out"=w210:refnum<vi>)  [unwired: 5 in]
                n88 = call <vilib>:"Rotate X-axis.vi"("angle unit"=w201, "Relative?"=w211, "error in (no error)"=w209, "angle"=w203, "Scene Object In"=w210) -> ("error out"=w208:errorcluster, "Scene Object Out"=w207:refnum<vi>)  [unwired: 5 in]
                n89 = call <vilib>:"Rotate Z-axis.vi"("angle unit"=w201, "Relative?"=w211, "error in (no error)"=w208, "angle"=w202, "Scene Object In"=w207) -> ("error out"=w199:errorcluster, "Scene Object Out"=w200:refnum<vi>)  [unwired: 5 in]
              }
              frame 11 {
                w225 = TRUE ("Relative?")
                n90 = call <vilib>:"Rotate Z-axis.vi"("angle unit"=w215, "Relative?"=FALSE, "error in (no error)"=w219, "angle"=w217, "Scene Object In"=w220) -> ("error out"=w223:errorcluster, "Scene Object Out"=w224:refnum<vi>)  [unwired: 5 in]
                n91 = call <vilib>:"Rotate Y-axis.vi"("angle unit"=w215, "Relative?"=w225, "error in (no error)"=w223, "angle"=w218, "Scene Object In"=w224) -> ("error out"=w222:errorcluster, "Scene Object Out"=w221:refnum<vi>)  [unwired: 5 in]
                n92 = call <vilib>:"Rotate Z-axis.vi"("angle unit"=w215, "Relative?"=w225, "error in (no error)"=w222, "angle"=w216, "Scene Object In"=w221) -> ("error out"=w213:errorcluster, "Scene Object Out"=w214:refnum<vi>)  [unwired: 5 in]
              }
            }
            n93 = call <vilib>:"Set Translation.vi"("error in (no error)"=w48, "Translation"=w49, "Scene Object"=w47) -> ()  [unwired: 7 in, 2 out]
          }
          frame True {
            w396 = -50.0 ("element")
            w448 = 100 ("dimension size")
            (unwired) "world32k.bmp" ("name or relative path")
            w450 = sgl 1.0 ("Row Interval")
            # "Initial P ECEF"
            # "Branco"
            # "Cria o frame do corpo"
            # "Cria o frame de navegação"
            # "This loads the texture map and\nreadies it to use on the ground."
            # "Use the random height matrix\nto generate a height grid."
            n94 = disable-structure shown="Disabled" {
              disable-tunnel: [w454 _] -> w442
              disable-tunnel: [w453 _] -> w434
              frame Disabled {
                n95 = Strip Path(path=path "world32k.bmp") -> (stripped path=w451:path)  [unwired: 1 out]
                n96 = call <vilib>:"Read PNG File.vi"("path to PNG file"=w451) -> ("error out"=w453:errorcluster, "image data"=w454:T8)  [unwired: 1 in, 8 out]
              }
              frame Enabled {
              }
            }
            n97 = Initialize Array(0.0 ("element"), w448, w448) -> (w446:dbl[][])
            n98 = call <vilib>:"Create Height Field.vi"("Column Interval"=w450, "Row Interval"=w450, "Data"=w446) -> ("error out"=w432:errorcluster, "New Height Field Refnum"=w441:refnum<vi>)  [unwired: 1 in, 6 out]
            n99 = call-poly <vilib>:"Create Object.vi"("error in (no error)"=w432, 10:w441, "Name"="Base") -> ("error out"=w433:errorcluster, "Scene:New Object"=w443:refnum<vi>)  [unwired: 7 in]
            n100 = Merge Errors(w433, w434) -> (w397:errorcluster)
            n101 = call-poly <vilib>:"Apply Texture.vi"("Horizontal Wrap Mode"=enum16{"Clamp", "Repeat"}."Repeat", "error in (no error)"=w397, "Apply Mode"=T5."As a Decal", "Image Data"=w442, "Scene Object In"=w443) -> ("error out"=w435:errorcluster, "Scene Object Out"=w445:refnum<vi>)  [unwired: 5 in]
            n102 = Bundle("element"=w396, "element"=w396, "element"=50.0) -> (w449:T9)  [unwired: 1 out]
            n103 = call <vilib>:"Set Translation.vi"("error in (no error)"=w435, "Translation"=w449, "Scene Object"=w445) -> ("error out"=w436:errorcluster, "Translated Object"=w439:refnum<vi>)  [unwired: 7 out]
            n104 = call-poly <vilib>:"Create Object.vi"("error in (no error)"="error in (no error)", "Name"="world") -> ("error out"=w437:errorcluster, "Scene:New Object"=w438:refnum<vi>)  [unwired: 8 in]
            n105 = disable-structure shown="Disabled" {
              disable-tunnel: w439 -> [w472 _]
              disable-tunnel: w438 -> [w471 w473]
              disable-tunnel: w437 -> [w470 w474]
              disable-tunnel: w436 -> [w468 _]
              disable-tunnel: [w456 w474] -> w415
              disable-tunnel: [w455 w473] -> w414
              frame Disabled {
                w467 = sgl 0.0 ("A")
                # "Underneath Clipping\nPlane: z = 0"
                n106 = Merge Errors(w470, w468) -> (w469:errorcluster)
                n107 = call-poly <vilib>:"Add Object.vi"("error in (no error)"=w469, "New Object In"=w472, "Scene Object In"=w471) -> ("error out"=w457:errorcluster, "Scene Object Out"=w458:refnum<vi>)  [unwired: 7 in]
                n108 = Bundle By Name(cluster=cluster{"A":sgl, "B":sgl, "C":sgl, "D":sgl} {"A"=0.0, "B"=0.0, "C"=0.0, "D"=0.0} ("Plane"), "A"=w467, "B"=w467, "C"=sgl 1.0 ("B"), "D"=sgl 0.01 ("B")) -> (w464:cluster{"A":sgl, "B":sgl, "C":sgl, "D":sgl})
                n109 = call <vilib>:"Create Clip Plane.vi"("error in (no error)"=w457, "Number"=0, "Plane"=w464) -> ("error out"=w460:errorcluster, "New Clip Plane Refnum"=w462:refnum<vi>)  [unwired: 7 out]
                n110 = call-poly <vilib>:"Set Clip Plane.vi"("error in (no error)"=w460, "Clip Plane State"=enum16{"Inherit Value", "Off", "On"}."Off", "Clip Plane Refnum In"=w462, "Scene Object In"=w458) -> ("error out"=w456:errorcluster, "Scene Object Out"=w455:refnum<vi>)  [unwired: 6 in]
              }
              frame Enabled {
              }
            }
            n111 = call <vilib>:"Create 3D Axis.vi"("Axis label?"=TRUE, "Color"=T6 {"Red"=1.0, "Green"=1.0, "Blue"=1.0, "Alpha"=1.0}, "Length"=sgl 1.0 ("Radius"), "Name"="N-Frame") -> ("error out"=w407:errorcluster, "New Object Refnum"=w406:refnum<vi>)  [unwired: 6 in]
            n112 = call <vilib>:"Create 3D Axis.vi"("Axis label?"=TRUE, "Color"=T6 {"Red"=0.0, "Green"=1.0, "Blue"=0.0, "Alpha"=1.0}, "Length"=sgl 1.0 ("Radius"), "Name"="B-Frame") -> ("error out"=w416:errorcluster, "New Object Refnum"=w417:refnum<vi>)  [unwired: 6 in]
            n113 = call-poly <vilib>:"Create Object.vi"("Name"="Corpo") -> ("error out"=w410:errorcluster, "Scene:New Object"=w411:refnum<vi>)  [unwired: 9 in]
            n114 = call <vilib>:"Set Translation.vi"("error in (no error)"=w410, "Translation"=cluster{"X":sgl, "Y":sgl, "Z":sgl} {"X"=0.0, "Y"=0.0, "Z"=0.0}, "Scene Object"=w411) -> ("error out"=w413:errorcluster, "Translated Object"=w412:refnum<vi>)  [unwired: 7 out]
            n115 = Merge Errors(w413, w416) -> (w420:errorcluster)
            n116 = call-poly <vilib>:"Add Object.vi"("error in (no error)"=w420, "New Object In"=w417, "Scene Object In"=w412) -> ("error out"=w418:errorcluster, "Scene Object Out"=w419:refnum<vi>)  [unwired: 7 in]
            n117 = call <vilib>:"Set Translation.vi"("error in (no error)"=w407, "Translation"=cluster{"X":sgl, "Y":sgl, "Z":sgl} {"X"=0.0, "Y"=0.0, "Z"=0.0}, "Scene Object"=w406) -> ("error out"=w405:errorcluster, "Translated Object"=w404:refnum<vi>)  [unwired: 7 out]
            n118 = Merge Errors(w415, w418) -> (w430:errorcluster)
            n119 = call-poly <vilib>:"Add Object.vi"("error in (no error)"=w430, "New Object In"=w419, "Scene Object In"=w414) -> ("error out"=w424:errorcluster, "Scene Object Out"=w427:refnum<vi>)  [unwired: 7 in]
            n120 = Merge Errors(w424, w405) -> (w423:errorcluster)
            n121 = call-poly <vilib>:"Add Object.vi"("error in (no error)"=w423, "New Object In"=w404, "Scene Object In"=w427) -> ("Scene Object Out"=w402:refnum<vi>)  [unwired: 7 in, 1 out]
          }
        }
        "3D Picture Control" <- w21
      }
      frame Enabled {
      }
    }
    n122 = shared-variable "NI-PXI8106\\Library 1.lvlib\\t"() -> (→"time[s]":dbl)  [unwired: 1 in, 1 out]
    n123 = shared-variable "NI-PXI8106\\Library 1.lvlib\\Run_SIM"("Run_SIM") -> ()  [unwired: 1 in, 1 out]
    n124 = shared-variable "NI-PXI8106\\Library 1.lvlib\\Stop_SIM"("stop Host") -> ()  [unwired: 1 in, 1 out]
    n125 = shared-variable ".\\Library 1.lvlib\\Sim_logdata"() -> (w11:dbl[])  [unwired: 1 in, 1 out]
    n126 = disable-structure shown="Disabled" {
      frame Disabled {
        n127 = shared-variable "My Computer\\Library 1.lvlib\\TVA_Address CRC Fault"() -> (w15:bool)  [unwired: 1 in, 1 out]
        n128 = disable-structure shown="Disabled" {
          disable-tunnel: [w19 _] -> w18
          frame Disabled {
            n129 = shared-variable "My Computer\\Library 1.lvlib\\Variable"() -> (w19:bool)  [unwired: 1 in, 1 out]
          }
          frame Enabled {
          }
        }
        "CRC data fault" <- w18
        n130 = Boolean To (0,1)(Boolean=w18) -> (0, 1=w17:i16)
        n131 = Boolean To (0,1)(Boolean=w15) -> (0, 1=w16:i16)
        n132 = To Double Precision Float(number=w17) -> ()  [unwired: 1 out]
        n133 = To Double Precision Float(number=w16) -> ()  [unwired: 1 out]
      }
      frame Enabled {
      }
    }
    n134 = Index Array(array=w11, index #1=0 ("index"), index #2=1 ("index")) -> (element #1=→"element":dbl)  [unwired: 31 in, 32 out]
    "Sim_Stopped" <- "stop Host"
  }
  n135 = case shown="\"CRC TVA\"" "Tab Control" {
    frame "Attitude Euler Angles" {
    }
    frame "Body Rates" {
    }
    frame "Body Accel" {
    }
    frame "Malpha/ Mbeta" {
    }
    frame "AoA" {
    }
    frame "ACT_b angles" {
    }
    frame "Oil Consumption" {
    }
    frame "Bending Moments" {
    }
    frame "CRC TVA" {
    }
    frame "Attitude Quaternions" {
    }
    frame "Velocity" {
    }
    frame "Position" {
    }
    frame "Attitude Comparison" {
    }
  }
  n136 = disable-structure shown="Disabled" {
    frame Disabled {
      n137 = Bundle() -> (w529:cluster{void, void})  [unwired: 3 in]
      n138 = Bundle() -> (w530:cluster{void, void})  [unwired: 3 in]
      n139 = Bundle() -> (w480:cluster{void, void})  [unwired: 3 in]
      n140 = Bundle() -> (w479:cluster{void, void}, w478)  [unwired: 2 in]
      n141 = Bundle() -> (w481:cluster{void, void})  [unwired: 3 in]
      n142 = Bundle() -> (→"Oil Consumption":cluster{void, void})  [unwired: 3 in]
      n143 = Bundle() -> (w522:cluster{void, void})  [unwired: 3 in]
      n144 = Bundle() -> (w523:cluster{void, void})  [unwired: 3 in]
      n145 = Bundle() -> (w524:cluster{void, void})  [unwired: 3 in]
      n146 = Bundle() -> (w527:cluster{void, void})  [unwired: 3 in]
      n147 = Bundle() -> (w526:cluster{void, void})  [unwired: 3 in]
      n148 = Bundle() -> (w525:cluster{void, void})  [unwired: 3 in]
      n149 = Bundle() -> (w519:cluster{void, void})  [unwired: 3 in]
      n150 = Bundle() -> (w520:cluster{void, void})  [unwired: 3 in]
      n151 = Bundle() -> (w521:cluster{void, void})  [unwired: 3 in]
      n152 = Bundle() -> (w517:cluster{void, void})  [unwired: 3 in]
      n153 = Bundle() -> (w514:cluster{void, void}, w491)  [unwired: 2 in]
      n154 = Bundle() -> (w515:cluster{void, void}, w489)  [unwired: 2 in]
      n155 = Bundle() -> (w516:cluster{void, void}, w488)  [unwired: 2 in]
      n156 = Bundle() -> (w483:cluster{void, void})  [unwired: 3 in]
      n157 = Bundle() -> (w482:cluster{void, void})  [unwired: 3 in]
      n158 = Bundle() -> (w509:cluster{void, void})  [unwired: 3 in]
      n159 = Bundle() -> (w512:cluster{void, void})  [unwired: 3 in]
      n160 = Bundle() -> (w511:cluster{void, void})  [unwired: 3 in]
      n161 = Bundle() -> (w505:cluster{void, void})  [unwired: 3 in]
      n162 = Bundle() -> (w507:cluster{void, void})  [unwired: 3 in]
      n163 = Bundle() -> (w508:cluster{void, void})  [unwired: 3 in]
      n164 = Bundle() -> (w504:cluster{void, void})  [unwired: 3 in]
      n165 = Bundle() -> (w503:cluster{void, void})  [unwired: 3 in]
      n166 = Bundle() -> (w500:cluster{void, void})  [unwired: 3 in]
      n167 = Bundle() -> (w501:cluster{void, void})  [unwired: 3 in]
      n168 = Bundle() -> (w498:cluster{void, void})  [unwired: 3 in]
      n169 = Bundle() -> (w497:cluster{void, void})  [unwired: 3 in]
      n170 = Bundle() -> (w492:cluster{void, void})  [unwired: 3 in]
      n171 = Bundle() -> (w493:cluster{void, void}, w475)  [unwired: 2 in]
      n172 = Bundle() -> (w487:cluster{void, void})  [unwired: 3 in]
      n173 = Bundle() -> (w486:cluster{void, void}, w476)  [unwired: 2 in]
      n174 = Bundle() -> (w485:cluster{void, void})  [unwired: 3 in]
      n175 = Bundle() -> (w484:cluster{void, void}, w477)  [unwired: 2 in]
      n176 = Build Array(w529, w530) -> ()  [unwired: 1 out]
      n177 = Build Array(w522, w523, w524) -> (→"Position":cluster{void, void}[])
      n178 = Build Array(w519, w520, w521, w517) -> (→"Quaternions":cluster{void, void}[])
      n179 = Build Array(w509, w512, w511) -> (→"Body Rates":cluster{void, void}[])
      n180 = Build Array(w505, w507, w508) -> (→"Body Accelerations":cluster{void, void}[])
      n181 = Build Array(w504, w503) -> (→"Malpha/ Mbeta":cluster{void, void}[])
      n182 = Build Array(w500, w501) -> (→"Angles of attack":cluster{void, void}[])
      n183 = Build Array(w498, w497) -> (→"ACT_b_angles":cluster{void, void}[])
      n184 = Build Array(w514, w515, w516, w483, w482) -> (→"Euler Angles":cluster{void, void}[])
      n185 = Build Array(w492, w493, w487, w486, w485, w484) -> (→"Euler Angles 2":cluster{void, void}[])
      n186 = Build Array(w527, w526, w525, w480, w479, w481) -> (→"Velocity":cluster{void, void}[])
    }
    frame Enabled {
    }
  }
